vi "State6-Straighten.vi"(10 "Numeric 2":dbl, 11 "Numeric":dbl) -> (1 "Cluster":T2, 2 "Front/Back 2":enum16{"Forward", "Backward", "Stop"}(ring), 3 "Left/Right":enum16{"Left", "Right", "Stop"}(ring), 4 "Enum":T1, 5 "Left/Right Speed":u32)   [LabVIEW 2014]
uses:
  FPGA Bitfiles/Parking States Indicators.ctl
  FPGA Bitfiles/Parking States.ctl
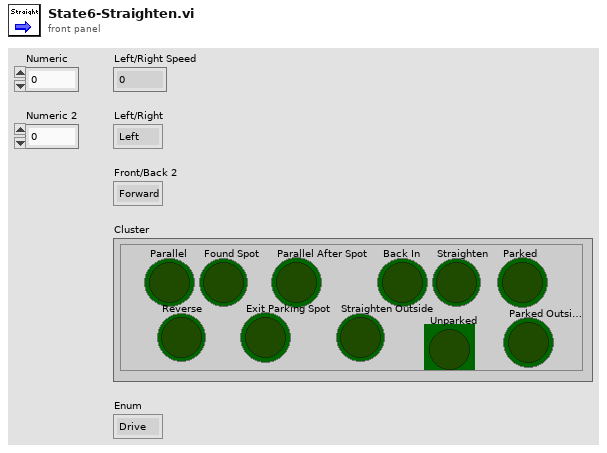
[diagram p1: front panel]
types:
  T1 = typedef "Parking States.ctl" = enum16{"Drive", "Parallel", "Found Spot", "Parallel After Spot", "Back In", "Straighten", "Parked", "Reverse", "Exit Parking Spot", "Straighten Outside", "Unparked", "Parked Outside"}
  T2 = typedef "Parking States Indicators.ctl" = cluster{"Parallel":bool, "Found Spot":bool, "Parallel After Spot":bool, "Back In":bool, "Straighten":bool, "Parked":bool, "Reverse":bool, "Exit Parking Spot":bool, "Straighten Outside":bool, "Unparked":bool, "Parked Outside":bool}
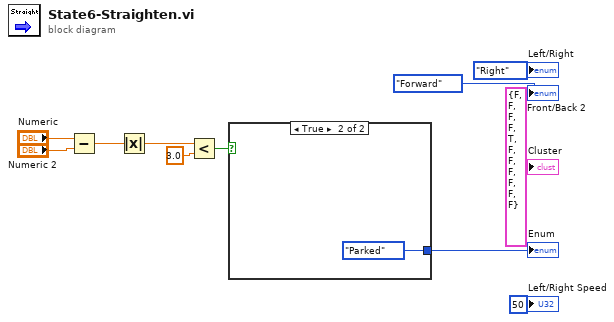
[diagram p0: block diagram]
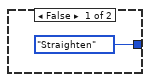
[diagram p2: hidden frame]
diagram:
  n1 = Subtract(x="Numeric", y="Numeric 2") -> (x-y=w5:dbl)
  n2 = Absolute Value(x=w5) -> (abs(x)=w6:dbl)
  n3 = Less?(x=w6, y=3.0) -> (x < y?=w8:bool)
  n4 = case shown="True" w8 {
    tunnel: [Parking_States."Straighten" Parking_States."Parked"] -> w2
    frame False {
    }
    frame True {
    }
  }
  "Enum" <- w2
  "Front/Back 2" <- enum16{"Forward", "Backward", "Stop"}."Forward" ("Front/Back 2")
  "Cluster" <- T2 {"Parallel"=FALSE, "Found Spot"=FALSE, "Parallel After Spot"=FALSE, "Back In"=FALSE, "Straighten"=TRUE, "Parked"=FALSE, "Reverse"=FALSE, "Exit Parking Spot"=FALSE, "Straighten Outside"=FALSE, "Unparked"=FALSE, "Parked Outside"=FALSE} ("Cluster")
  "Left/Right Speed" <- u32 50 ("Left/Right Speed")
  "Left/Right" <- enum16{"Left", "Right", "Stop"}."Right" ("Left/Right")
